vi "Software Update HCC Search and Build Array.vi"(6 "Search Expression":string, 7 "New Software Path":path, 8 "Error In":errorcluster, 10 "Input Path":path, 11 "Filenames Input":string[](array[string])) -> (0 "Error Out":errorcluster, 1 "Software Version":string, 2 "Archive Folder":path, 3 "Output Path":path[](array[path]), 4 "Target Folder":path, 5 "Skip if Revision is the Same":bool)   [LabVIEW 2016]
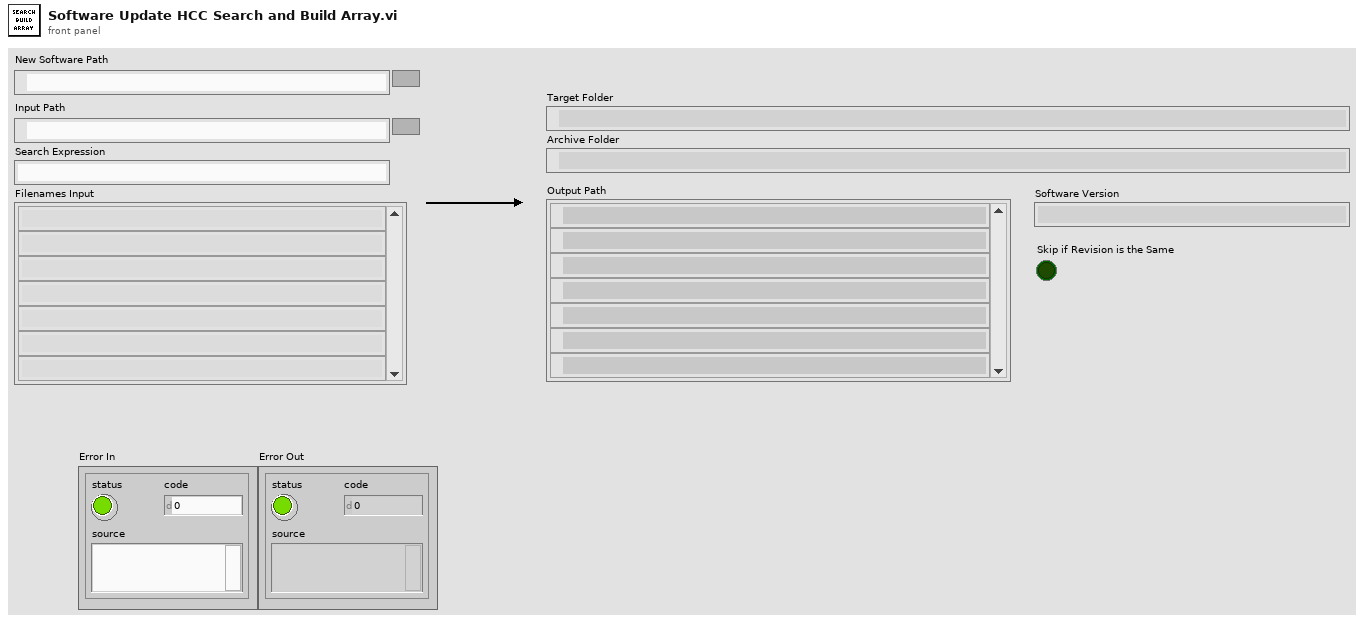
[diagram p1: front panel]
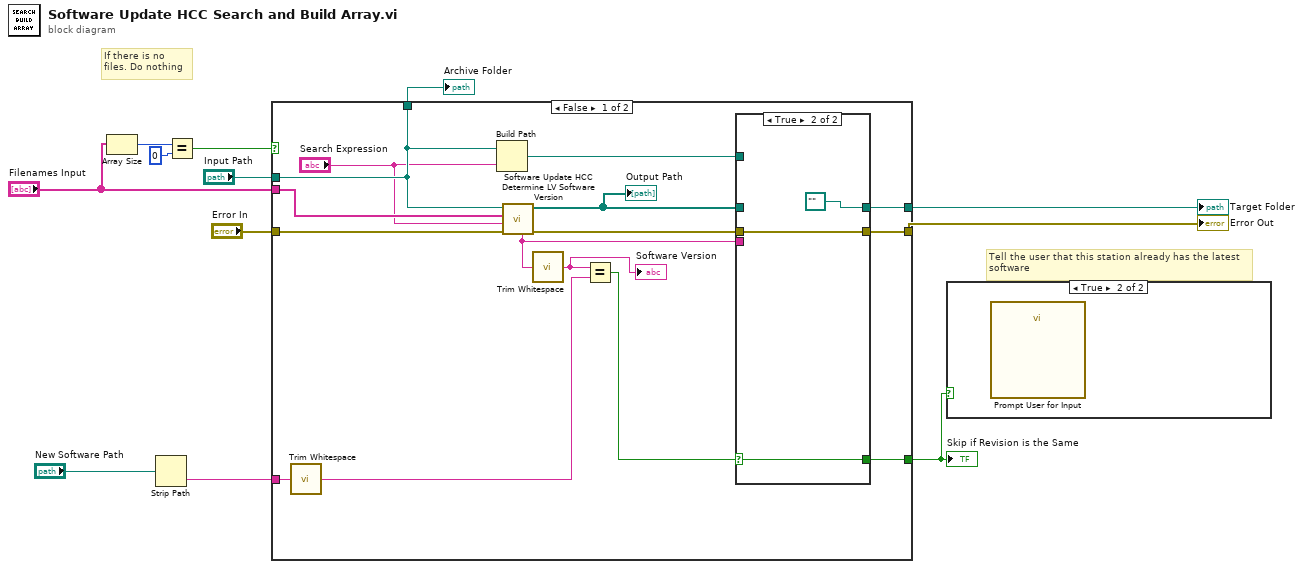
[diagram p0: block diagram]
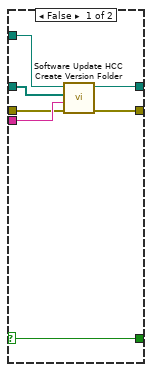
[diagram p3: hidden frame]
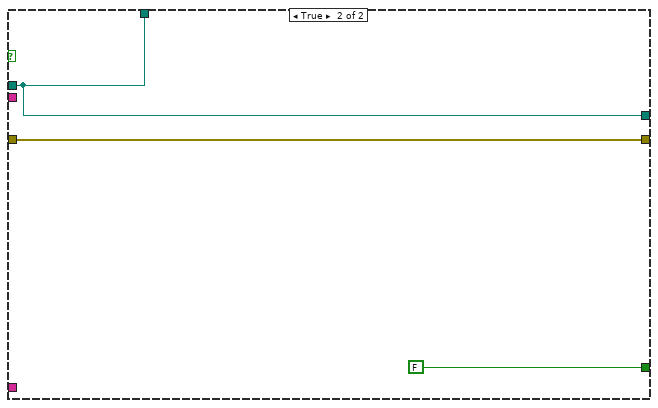
[diagram p4: hidden frame]
diagram:
  # "Tell the user that this station already has the latest\nsoftware"
  # "If there is no \nfiles. Do nothing"
  n1 = Array Size(array="Filenames Input") -> (size(s)=w11:i32)
  n2 = Strip Path(path="New Software Path") -> (name=w4:string)  [unwired: 1 out]
  n3 = Equal?(x=w11, y=0) -> (x = y?=w9:bool)
  n4 = case shown="False" w9 {
    tunnel: "Filenames Input" -> [w27 _]
    tunnel: "Input Path" -> [w25 w40]
    tunnel: [w25 w40] -> w7
    tunnel: [w26 w40] -> w6
    tunnel: w4 -> [w21 _]
    tunnel: [w17 FALSE] -> w3
    tunnel: "Error In" -> [w16 w38]
    tunnel: [w15 w38] -> w1
    frame False {
      n5 = call <vilib>:"Trim Whitespace.vi"("string"=w21) -> ("trimmed string"=w19:string)  [unwired: 1 in]
      n6 = Build Path(base path=w25, name or relative path="Search Expression") -> (appended path=w24:path)
      n7 = call "Software Update HCC Determine LV Software Version.vi"("Error In"=w16, "Search Expression in"="Search Expression", "Filenames Input"=w27, "Input Path"=w25) -> ("Error Out"=w14:errorcluster, "Output Path"=w22:path[], "Software Version"=w20:string)  [unwired: 5 in]
      "Output Path" <- w22
      n8 = call <vilib>:"Trim Whitespace.vi"("string"=w20) -> ("trimmed string"=w13:string)  [unwired: 1 in]
      "Software Version" <- w13
      n9 = Equal?(x=w13, y=w19) -> (x = y?=w18:bool)
      n10 = case shown="True" w18 {
        selector: w18 -> [w30 w37]
        tunnel: [w34 path "" ("Target Folder")] -> w26
        tunnel: w24 -> [w33 _]
        tunnel: w22 -> [w32 _]
        tunnel: w20 -> [w31 _]
        tunnel: [w30 w37] -> w17
        tunnel: [w29 w35] -> w15
        tunnel: w14 -> [w28 w35]
        frame False {
          n11 = call "Software Update HCC Create Version Folder.vi"("Error In"=w28, "Software Version"=w31, "Output Path"=w32, "Archive Software By Software Type (Ex: C:\\Newfi Exe\\Exe5\\Archive\\Newfi\\)"=w33) -> ("Error Out"=w29:errorcluster, "Target Folder"=w34:path)  [unwired: 6 in]
        }
        frame True {
        }
      }
    }
    frame True {
    }
  }
  "Archive Folder" <- w7
  "Target Folder" <- w6
  "Skip if Revision is the Same" <- w3
  "Error Out" <- w1
  n12 = case shown="True" w3 {
    frame False {
    }
    frame True {
      n13 = call "Prompt User for Input"() -> ()  [unwired: 18 in, 2 out]
    }
  }
